vi "Write Config Unitest.vi"(8 "error in (no error)":errorcluster, 11 "main ref":T1) -> (0 "error out":errorcluster)   [LabVIEW 2025]
uses:
  controls/LAB-IQ UI Data.ctl
  Config file  FGV Unitest enum.ctl
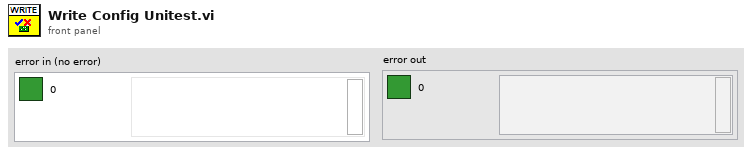
[diagram p1: front panel]
types:
  T1 = typedef "LAB-IQ UI Data.ctl" = cluster{"Main Home Screen":cluster{"GUI":refnum<vi>, "Platform Settings":refnum<vi>, "Configure":refnum<vi>, "Home":refnum<vi>, "EXIT":refnum<vi>, "service 2":refnum<vi>, "MainPage":refnum<vi>, "Analysis":refnum<vi>}, "Platform Settings":cluster{"mm/s  Surge":refnum<vi>, "Update Surge Speed":refnum<vi>, "Drive Error":refnum<vi>, "Disable Axis Jog Soft Limits":refnum<vi>, "mm/s  Sway":refnum<vi>, "Sway and Surge COM Status":refnum<vi>, "Heave COM Status":refnum<vi>, "Enable Platform":refnum<vi>, "Surge Forward Main":refnum<vi>, "Sway Right Main":refnum<vi>, "Sway Left Main":refnum<vi>, "Heave Down Main":refnum<vi>, "Heave Up main":refnum<vi>, "Update Sway Speed":refnum<vi>, "Update Heave Speed":refnum<vi>, "mm/s Heave":refnum<vi>, "mm/sec":refnum<vi>, "mm":refnum<vi>, "Surge Backward Main":refnum<vi>}, "Analysis Screen":cluster{"Analysis Home":refnum<vi>, "Surface Analysis":refnum<vi>, "Imaging":refnum<vi>, "Image Analysis":refnum<vi>, "Post Analysis":refnum<vi>}, "Config Screen":cluster{"Select Load Head":refnum<vi>, "Notes :":refnum<vi>, "FILE":refnum<vi>, "Sample ID :":refnum<vi>, "Operator ID :":refnum<vi>, "Operator Name :":refnum<vi>, "Auto":refnum<vi>}, "Motion Module":cluster{"zNL":refnum<vi>, "NL disp":refnum<vi>, "Rotary Tab":refnum<vi>, "Motion Direction:  3":refnum<vi>, "E.Velocity 2":refnum<vi>, "e.v/ssr 2":refnum<vi>, "Enter Fixed E.Velocity 2":refnum<vi>, "Enter Final SRR 2":refnum<vi>, "Enter initial SRR 2":refnum<vi>, "Enter Fixed SRR 2":refnum<vi>, "Enter the Final E.Velocity (m/s) 2":refnum<vi>, "Enter initial E.Velocity (m/s) 2":refnum<vi>, "Final Speed (RPM) 3":refnum<vi>, "Initial Speed (RPM) 2":refnum<vi>, "Enter the Final Velocity (m/s) 3":refnum<vi>, "Enter initial Velocity (m/s)  3":refnum<vi>, "Ramp Up 2":refnum<vi>, "TEST SELECTION":refnum<vi>, "SPEED SELECTION : ":refnum<vi>, "Angular Oscillation Set":refnum<vi>, "Traction":refnum<vi>, "Step Speed":refnum<vi>, "StepTable For Load-Speed":refnum<vi>, "StepTable For Speed":refnum<vi>, "Surge Forward MM":refnum<vi>, "Surge Backward MM":refnum<vi>, "M3 Image":refnum<vi>, "String 39":refnum<vi>, "Sway Left MM":refnum<vi>, "Sway Right MM":refnum<vi>, "Disable Axis Jog Soft Limits":refnum<vi>, "mm":refnum<vi>, "Heave Down MM":refnum<vi>, "Heave Up MM":refnum<vi>, "Wear Track Diameter (mm)":refnum<vi>, "Set WTD":refnum<vi>, "HomeScratch":refnum<vi>, "HomeRot":refnum<vi>, "PlaceModule":refnum<vi>, "Enter the Angle (Deg)":refnum<vi>, "Enter the Frequency (Hz)":refnum<vi>, "Motion Mode:":refnum<vi>, "LR Sway":refnum<vi>, "Rot Hor":refnum<vi>, "Scratch":refnum<vi>, "LR Cam":refnum<vi>, "MMBack":refnum<vi>, "MMNext":refnum<vi>, "Rot Ver":refnum<vi>, "Rotary Module Selection":refnum<vi>, "calculate rotary":refnum<vi>, "SPEED SELECTION : rotary":refnum<vi>, "Import 2":refnum<vi>, "Save 2":refnum<vi>, "File Path :  2":refnum<vi>, "String 45":refnum<vi>, "StepTable For Speed 3":refnum<vi>, "Enter the Speed(mm/sec)":refnum<vi>, "Enter the Speed(RPM)":refnum<vi>, "Enter Scratch Speed (mm/s):":refnum<vi>, "SwaySpeed Set":refnum<vi>, "Scartch Offset":refnum<vi>, "Motion type:":refnum<vi>, "HomeScratch 2":refnum<vi>, "Enter Scratch length (mm):":refnum<vi>, "Wear Track Diameter":refnum<vi>, "Rotary Speed Exced":refnum<vi>, "Scratch Mode":refnum<vi>, "No of Scratch":refnum<vi>}, "Environmental control":cluster{"Humidity  Status  3":refnum<vi>, "Low Temp  Status  2":refnum<vi>, "TK4 status 2":refnum<vi>, "Stage Temperature":refnum<vi>, "Sample Temperature":refnum<vi>, "Humidity (Amb)":refnum<vi>, "Clear List":refnum<vi>, "Add to list":refnum<vi>, "Wear":refnum<vi>, "Vibration":refnum<vi>, "Humidity (Chamber)":refnum<vi>, "Temperature (Chamber)":refnum<vi>, "ECR ":refnum<vi>, "Temperature (Amb)":refnum<vi>, "Microphone":refnum<vi>, "Acoustic Emission 3":refnum<vi>, "SNext":refnum<vi>, "APBack":refnum<vi>, "Enter the Temperature (°C):":refnum<vi>, "Enter the Stage \nTemperature (°C):":refnum<vi>, "Enter the Humidity (%Rh):":refnum<vi>, "Low Temp":refnum<vi>, "High Temp":refnum<vi>, "Humidity":refnum<vi>, "Sensors Picked":refnum<vi>}, "About Screen":cluster{"Password":refnum<vi>, "Home Service":refnum<vi>, "Advanced Setting":refnum<vi>, "About Tab":refnum<vi>, "ECR Port:":refnum<vi>, "Ramp Port:":refnum<vi>, "Installation/Replacement completed":refnum<vi>, "Loahead":refnum<vi>, "Heave and Surge COM Port:":refnum<vi>, "Sway COM Port:":refnum<vi>, "Temp Modbus:":refnum<vi>, "Humidity Port:":refnum<vi>, "Edit Gain Constants":refnum<vi>, "Save Gain Constants":refnum<vi>}, "Main Screen":cluster{"Main Screen Tab":refnum<vi>, "Angle and Frequency":refnum<vi>, "Stroke (mm)":refnum<vi>, "Angle (Deg)":refnum<vi>, "Main Speed Tab":refnum<vi>, "MTM MOTOR DISPLAY":refnum<vi>, "Disc Speed (m/sec)":refnum<vi>, "Ball Speed (m/sec)":refnum<vi>, "Disc Speed (RPM)":refnum<vi>, "Ball Speed (RPM)":refnum<vi>, "SPEED TAB":refnum<vi>, "Speed (m/sec)":refnum<vi>, "Set Speed (m/sec)":refnum<vi>, "Speed (RPM)":refnum<vi>, "Set Speed":refnum<vi>, "Time Tab":refnum<vi>, "Time ( HH:MM:SS ) 2":refnum<vi>, "Test Duration":refnum<vi>, "Test Duration 4":refnum<vi>, "TEST CYCLE":refnum<vi>, "TOTAL CYCLES":refnum<vi>, "Set Load (N)":refnum<vi>, "Temp Tabs":refnum<vi>, "Heater":refnum<vi>, "TK4 status":refnum<vi>, "ChamberTemp":refnum<vi>, "SetTmp":refnum<vi>, "Controller  Status":refnum<vi>, "ChamberTemp 2":refnum<vi>, "SetTmp 2":refnum<vi>, "Controller  Status 2":refnum<vi>, "ChamberTemp 3":refnum<vi>, "SetTmp 3":refnum<vi>, "Cooling":refnum<vi>, "Load Communication":refnum<vi>, "Ambient \nTemperature":refnum<vi>, "HumCOMStatus":refnum<vi>, "Ambient\n Humidity":refnum<vi>, "Freq (Hz)":refnum<vi>, "Load En":refnum<vi>, "NLt":refnum<vi>, "zNL 2":refnum<vi>, "Humidity On":refnum<vi>, "humidity disp":refnum<vi>, "Set Humidity":refnum<vi>, "NL disp 2":refnum<vi>, "Humidity On 2":refnum<vi>, "humidity disp 2":refnum<vi>, "Set Humidity 2":refnum<vi>, "NL disp 3":refnum<vi>, "AppLoadSeq scratch":refnum<vi>, "Stop Scratch":refnum<vi>, "ClrLog":refnum<vi>, "Trip Log":refnum<vi>, "STOP":refnum<vi>, "Start Test":refnum<vi>, "Test status":refnum<vi>, "AR Led":refnum<vi>, "Data":refnum<vi>, "Health":refnum<vi>, "Sway COM Status":refnum<vi>, "Heave COM Status":refnum<vi>, "Grp Tab":refnum<vi>, "Sub Graph":refnum<vi>, "SD (mm)":refnum<vi>, "Siliding distance Reset Graph":refnum<vi>, "SDGp":refnum<vi>, "Humidity Reset Graph":refnum<vi>, "HumrGp":refnum<vi>, "Acoustic Emission (mV)":refnum<vi>, "Aqucostic Reset Graph":refnum<vi>, "gACQUOS":refnum<vi>, "ECR RESET":refnum<vi>, "ECR":refnum<vi>, "Temperature Reset":refnum<vi>, "Acoustic Emission (mV) 2":refnum<vi>, "Aqucostic Reset Graph 2":refnum<vi>, "gACQUOS 2":refnum<vi>, "ECR RESET 2":refnum<vi>, "ECR 2":refnum<vi>, "Temperature Reset 2":refnum<vi>, "Temperature (deg c)":refnum<vi>, "Speed Reset Graph":refnum<vi>, "Speed Tab":refnum<vi>, "MTM DISC  SPEED":refnum<vi>, "MTM BALL SPEED":refnum<vi>, "speed mm/sec":refnum<vi>, "Hymidity":refnum<vi>, "Humidity Disable trip":refnum<vi>, "CoF Trip  2":refnum<vi>, "Depth Trip":refnum<vi>, "Weart Deapth":refnum<vi>, "Depth Reset Graph":refnum<vi>, "Weart":refnum<vi>, "Depthz":refnum<vi>, "Depth (µm)":refnum<vi>, "WearGp":refnum<vi>, "NL Trip 2":refnum<vi>, "Load pid":refnum<vi>, "Load Disable Trip":refnum<vi>, "Load Reset Graph":refnum<vi>, "NL Display 4":refnum<vi>, "Main Chart 3":refnum<vi>, "BACK":refnum<vi>, "Depth Trip 2":refnum<vi>, "COF TRIP ":refnum<vi>, "Friction Force (N)":refnum<vi>, "FF Reset Graph":refnum<vi>, "FF Disable Trip":refnum<vi>, "FF TRIP":refnum<vi>, "COF Disable Trip":refnum<vi>, "COF Reset Graph":refnum<vi>, "Start Test Temp":refnum<vi>, "zFF":refnum<vi>, "Friction Force (N) Graph":refnum<vi>, "Coefficient of Friction":refnum<vi>, "Scratch Start Test":refnum<vi>, "FF Tab":refnum<vi>, "Cyclic Friction Force (N)":refnum<vi>, "CZ FF":refnum<vi>, "Cyclic Friction Force (N) Graph":refnum<vi>, "Cyclic Coefficient of Friction":refnum<vi>, "Cyclic FF TRIP":refnum<vi>, "Cyclic FF Disable Trip":refnum<vi>, "cyclic COF Disable Trip":refnum<vi>, "cyclic COF TRIP":refnum<vi>, "cyclic COF Reset Graph":refnum<vi>, "Cyclic FF Reset Graph":refnum<vi>, "Test Trip":refnum<vi>, "Multi Scratch Pass":refnum<vi>}, "Loading":cluster{"Indentation":refnum<vi>, "Reference Sample":refnum<vi>, "Load Cell Communication Slide":refnum<vi>, "com 3":refnum<vi>, "com":refnum<vi>, "DecaForce COM Status":refnum<vi>, "Update":refnum<vi>, "Clear 3":refnum<vi>, "seq":refnum<vi>, "Stribeck table":refnum<vi>, "Stribeck Table  For loading":refnum<vi>, "Loading Mode":refnum<vi>, "Enter the Final Load (N)":refnum<vi>, "Enter the CoF Trip":refnum<vi>, "Enter the Friction Force Trip":refnum<vi>, "Enter the Normal load Trip":refnum<vi>, "Enter the Load  (N)":refnum<vi>, "KiloForce":refnum<vi>, "DecaForce ":refnum<vi>, "MicroForce":refnum<vi>, "LHBack":refnum<vi>, "LHNext":refnum<vi>, "Enter the Loading Rate (N/min)":refnum<vi>, "Message":refnum<vi>, "Warning 2":refnum<vi>, "SSP 0.75":refnum<vi>, "SSP 0.5":refnum<vi>, "SSP 0.3":refnum<vi>, "Warning":refnum<vi>, "gui GIF":refnum<vi>, "Communication is established":refnum<vi>, "AppLoad 4":refnum<vi>, "Multipoint":refnum<vi>, "Load Selection":refnum<vi>}, "PID":cluster{"Ramp MulFac":refnum<vi>, "pulses LoadDiffRamp(2..10)":refnum<vi>, "PulseControlRamp(diff<=3N)":refnum<vi>, "SetLoadDeadband(%) Load(0-10N)":refnum<vi>, "PID gains out delay (microForce)":refnum<vi>, "Ramp":refnum<vi>, "Gain 2":refnum<vi>, "pulses LoadDiff(2..10)":refnum<vi>, "pulses LoadDiff(11..50)":refnum<vi>, "PulseControl(diff<=3N)":refnum<vi>, "SetLoadDeadband(%)  2":refnum<vi>, "Dummy Run":refnum<vi>, "Vertical load (N)":refnum<vi>, "AutoTune":refnum<vi>, "Offset 3 ":refnum<vi>, "apply load":refnum<vi>, "Offset  3":refnum<vi>, "apply load 2":refnum<vi>, "Enter ByPass Load":refnum<vi>, "reinit 3":refnum<vi>, "output range delay":refnum<vi>, "PID gains out delay":refnum<vi>, "Bypass Load":refnum<vi>, "pulsesSent":refnum<vi>, "pulses ":refnum<vi>, "actpid":refnum<vi>, "gFF Rot":refnum<vi>, "pulses LoadDiff(21..1000)":refnum<vi>, "Delay":refnum<vi>, "deadband":refnum<vi>}, "Config Parameters":cluster{"Tab Control 3":refnum<vi>, "Tab Control 19":refnum<vi>, "SAMPLES":refnum<vi>, "Re-initilaize":refnum<vi>, "Filter ON/OFF":refnum<vi>, "TracHomeSurgeOffsetCounts 10MM":refnum<vi>, "TracHomeSwayOffsetCounts 10MM":refnum<vi>, "Acoustic Emission:":refnum<vi>, "Apply Filter (FF)":refnum<vi>, "Filter% 2":refnum<vi>, "Apply Filter (Load)":refnum<vi>, "Filter% ":refnum<vi>, "Sway distance (mm)":refnum<vi>, "Surge distance (mm)":refnum<vi>, "DataSavingLoopDelay(ms)":refnum<vi>, "SAVE 2":refnum<vi>, "Enter Distance":refnum<vi>, "Sway Counts:":refnum<vi>, "Distance (mm): 3":refnum<vi>, "Surge Counts:":refnum<vi>, "Distance (mm): 2":refnum<vi>, "Distance (mm):":refnum<vi>, "Heave Counts:":refnum<vi>, "LRMHomeSurgeOffsetCounts":refnum<vi>, "LRMHomeSwayOffsetCounts":refnum<vi>, "TracHomeSurgeOffsetCounts 20MM":refnum<vi>, "TracHomeSwayOffsetCounts 20MM":refnum<vi>, "RotHomeSwayOffsetCounts":refnum<vi>, "RotHomeSurgeOffsetCounts":refnum<vi>, "Heave distance":refnum<vi>, "Zmm":refnum<vi>, "Heave Pulses/mm":refnum<vi>, "Surge Pulses/mm":refnum<vi>, "Sway Pulses/mm":refnum<vi>, "Heave Pitch":refnum<vi>, "Surge Pitch":refnum<vi>, "Sway Pitch":refnum<vi>, "Heave PPR":refnum<vi>, "Surge PPR":refnum<vi>, "Sway PPR":refnum<vi>, "Tab Control 5":refnum<vi>, "Tab Control 14":refnum<vi>, "Tab Control 26":refnum<vi>, "AE":refnum<vi>, "Heave Loop Delay":refnum<vi>, "Heave PID Speed":refnum<vi>, "Surge Jog Speed":refnum<vi>, "Heave Jog Speed":refnum<vi>, "Sway Loop Delay":refnum<vi>, "Sway PID Speed":refnum<vi>, "Sway Jog Speed":refnum<vi>}, "Loading Com Port":cluster{"ClearAll":refnum<vi>, "Mz(Nm)":refnum<vi>, "My(Nm)":refnum<vi>, "Mx(Nm)":refnum<vi>, "Save Dwell":refnum<vi>, "Mx ":refnum<vi>, "My ":refnum<vi>, "Mz":refnum<vi>, "Fx(N)":refnum<vi>, "Fy(N)":refnum<vi>, "Fz(N)":refnum<vi>, "ZeroAll":refnum<vi>, "Acq Delay (ms)":refnum<vi>, "Burst Delay (ms)":refnum<vi>, "model":refnum<vi>, "SN":refnum<vi>, "FFx(N)":refnum<vi>, "Sensor IP":refnum<vi>, "Port":refnum<vi>, "FFy(N)":refnum<vi>, "Load(N)":refnum<vi>, "delete Handle":refnum<vi>, "Create Handle":refnum<vi>, "ft_data":refnum<vi>, "ft_range":refnum<vi>, "ft_data 2":refnum<vi>, "stop 6":refnum<vi>, "running_flag":refnum<vi>, "ft_udp_handle":refnum<vi>, "get-data-return":refnum<vi>, "get-range-return":refnum<vi>, "zero-return":refnum<vi>, "filter-return":refnum<vi>, "initial-return":refnum<vi>, "deleteHandle-result":refnum<vi>, "Load Cell Temp":refnum<vi>}, "Heave AND Surge":cluster{"SURGE POSE":refnum<vi>, "error out Read":refnum<vi>, "HEAVE POSE":refnum<vi>, "State":refnum<vi>, "Homed":refnum<vi>, "Sequence ID":refnum<vi>, "error out Write":refnum<vi>, "faultCode":refnum<vi>, "Ack ID":refnum<vi>, "SPEED":refnum<vi>, "Distance":refnum<vi>, "Mode Command":refnum<vi>, "Heave and Surge Read":refnum<vi>, "Read Heave Temp":refnum<vi>, "Spare 15":refnum<vi>, "Spare 14":refnum<vi>, "Spare 13":refnum<vi>, "Spare 12":refnum<vi>, "Spare 11":refnum<vi>, "Spare 10":refnum<vi>, "Spare 9":refnum<vi>, "Spare 8":refnum<vi>, "Spare 7":refnum<vi>, "Spare 6":refnum<vi>, "Spare 5":refnum<vi>, "Spare 4":refnum<vi>, "Spare 2":refnum<vi>, "Spare 1":refnum<vi>, "Node Id":refnum<vi>, "Spare 3":refnum<vi>, "SPARE 4":refnum<vi>, "SPARE 3":refnum<vi>, "SPARE 2":refnum<vi>, "SPARE 1":refnum<vi>, "fwMajor":refnum<vi>, "fwMinor":refnum<vi>, "Manual Write":refnum<vi>, "Heave and Surge Write":refnum<vi>}, "New PID LOGIC":cluster{"Fine Tune Zone":refnum<vi>, "PID SDelay":refnum<vi>, "Max_pos_limit":refnum<vi>, "Min_pos_limit":refnum<vi>, "i_limit":refnum<vi>, "pct_scale":refnum<vi>, "Deadband":refnum<vi>, "Kd":refnum<vi>, "Ki":refnum<vi>, "Kp":refnum<vi>, "Current Position":refnum<vi>, "Set Load":refnum<vi>, "Current Load":refnum<vi>, "Pulse delta":refnum<vi>, "Init Step":refnum<vi>, "Max Step Linit":refnum<vi>}, "SWAY ":cluster{"fwMajor":refnum<vi>, "Homed":refnum<vi>, "Rotary POSE":refnum<vi>, "State":refnum<vi>, "SWAY POSE":refnum<vi>, "Ack ID":refnum<vi>, "faultCode":refnum<vi>, "Node Id":refnum<vi>, "fwMinor":refnum<vi>, "Spare 6":refnum<vi>, "Spare 5":refnum<vi>, "Spare 4":refnum<vi>, "Spare 3":refnum<vi>, "Spare 2":refnum<vi>, "Spare 1":refnum<vi>, "Spare 7":refnum<vi>, "SPARE  5":refnum<vi>, "error out Write  SWAY ":refnum<vi>, "error out Read SWAY ":refnum<vi>, "Manual Write SWAY ":refnum<vi>, "SWAY WRITE":refnum<vi>, "SPARE  4":refnum<vi>, "SPARE  3":refnum<vi>, "SPARE 2":refnum<vi>, "SPARE 1":refnum<vi>, "Spare 15":refnum<vi>, "Spare 14":refnum<vi>, "Spare 13":refnum<vi>, "Spare 12":refnum<vi>, "Spare 11":refnum<vi>, "Spare 9":refnum<vi>, "Spare 8":refnum<vi>, "SPEED":refnum<vi>, "Distance":refnum<vi>, "Mode Command":refnum<vi>, "Sequence ID":refnum<vi>, "SWAY READ":refnum<vi>, "Spare 10":refnum<vi>, "Read SWAY Temp":refnum<vi>}, "Analysis Screen":cluster{"Analysis Home":refnum<vi>, "Refresh 2":refnum<vi>, "MEAN 4":refnum<vi>, "SD 4":refnum<vi>, "VARIANCE 4":refnum<vi>, "MEAN  3":refnum<vi>, "SD  3":refnum<vi>, "VARIANCE  3":refnum<vi>, "MEAN 2":refnum<vi>, "SD  2":refnum<vi>, "VARIANCE 2":refnum<vi>, "MEAN":refnum<vi>, "SD":refnum<vi>, "VARIANCE":refnum<vi>, "File 4 Discription":refnum<vi>, "OPEN 4":refnum<vi>, "File Name 4":refnum<vi>, "OPEN 3":refnum<vi>, "File 3 Discription":refnum<vi>, "File Name 3":refnum<vi>, "Y-AXIS":refnum<vi>, "X-AXIS":refnum<vi>, "XY Graph":refnum<vi>, "File Name 2":refnum<vi>, "File Name 1":refnum<vi>, "OPEN 2":refnum<vi>, "OPEN 1":refnum<vi>, "File 1 Discription ":refnum<vi>, "File 2 Discription":refnum<vi>}}
  T2 = typedef "Config file  FGV Unitest enum.ctl" = enum16{"OPEN", "READ", "WRITE", "CLOSE"}
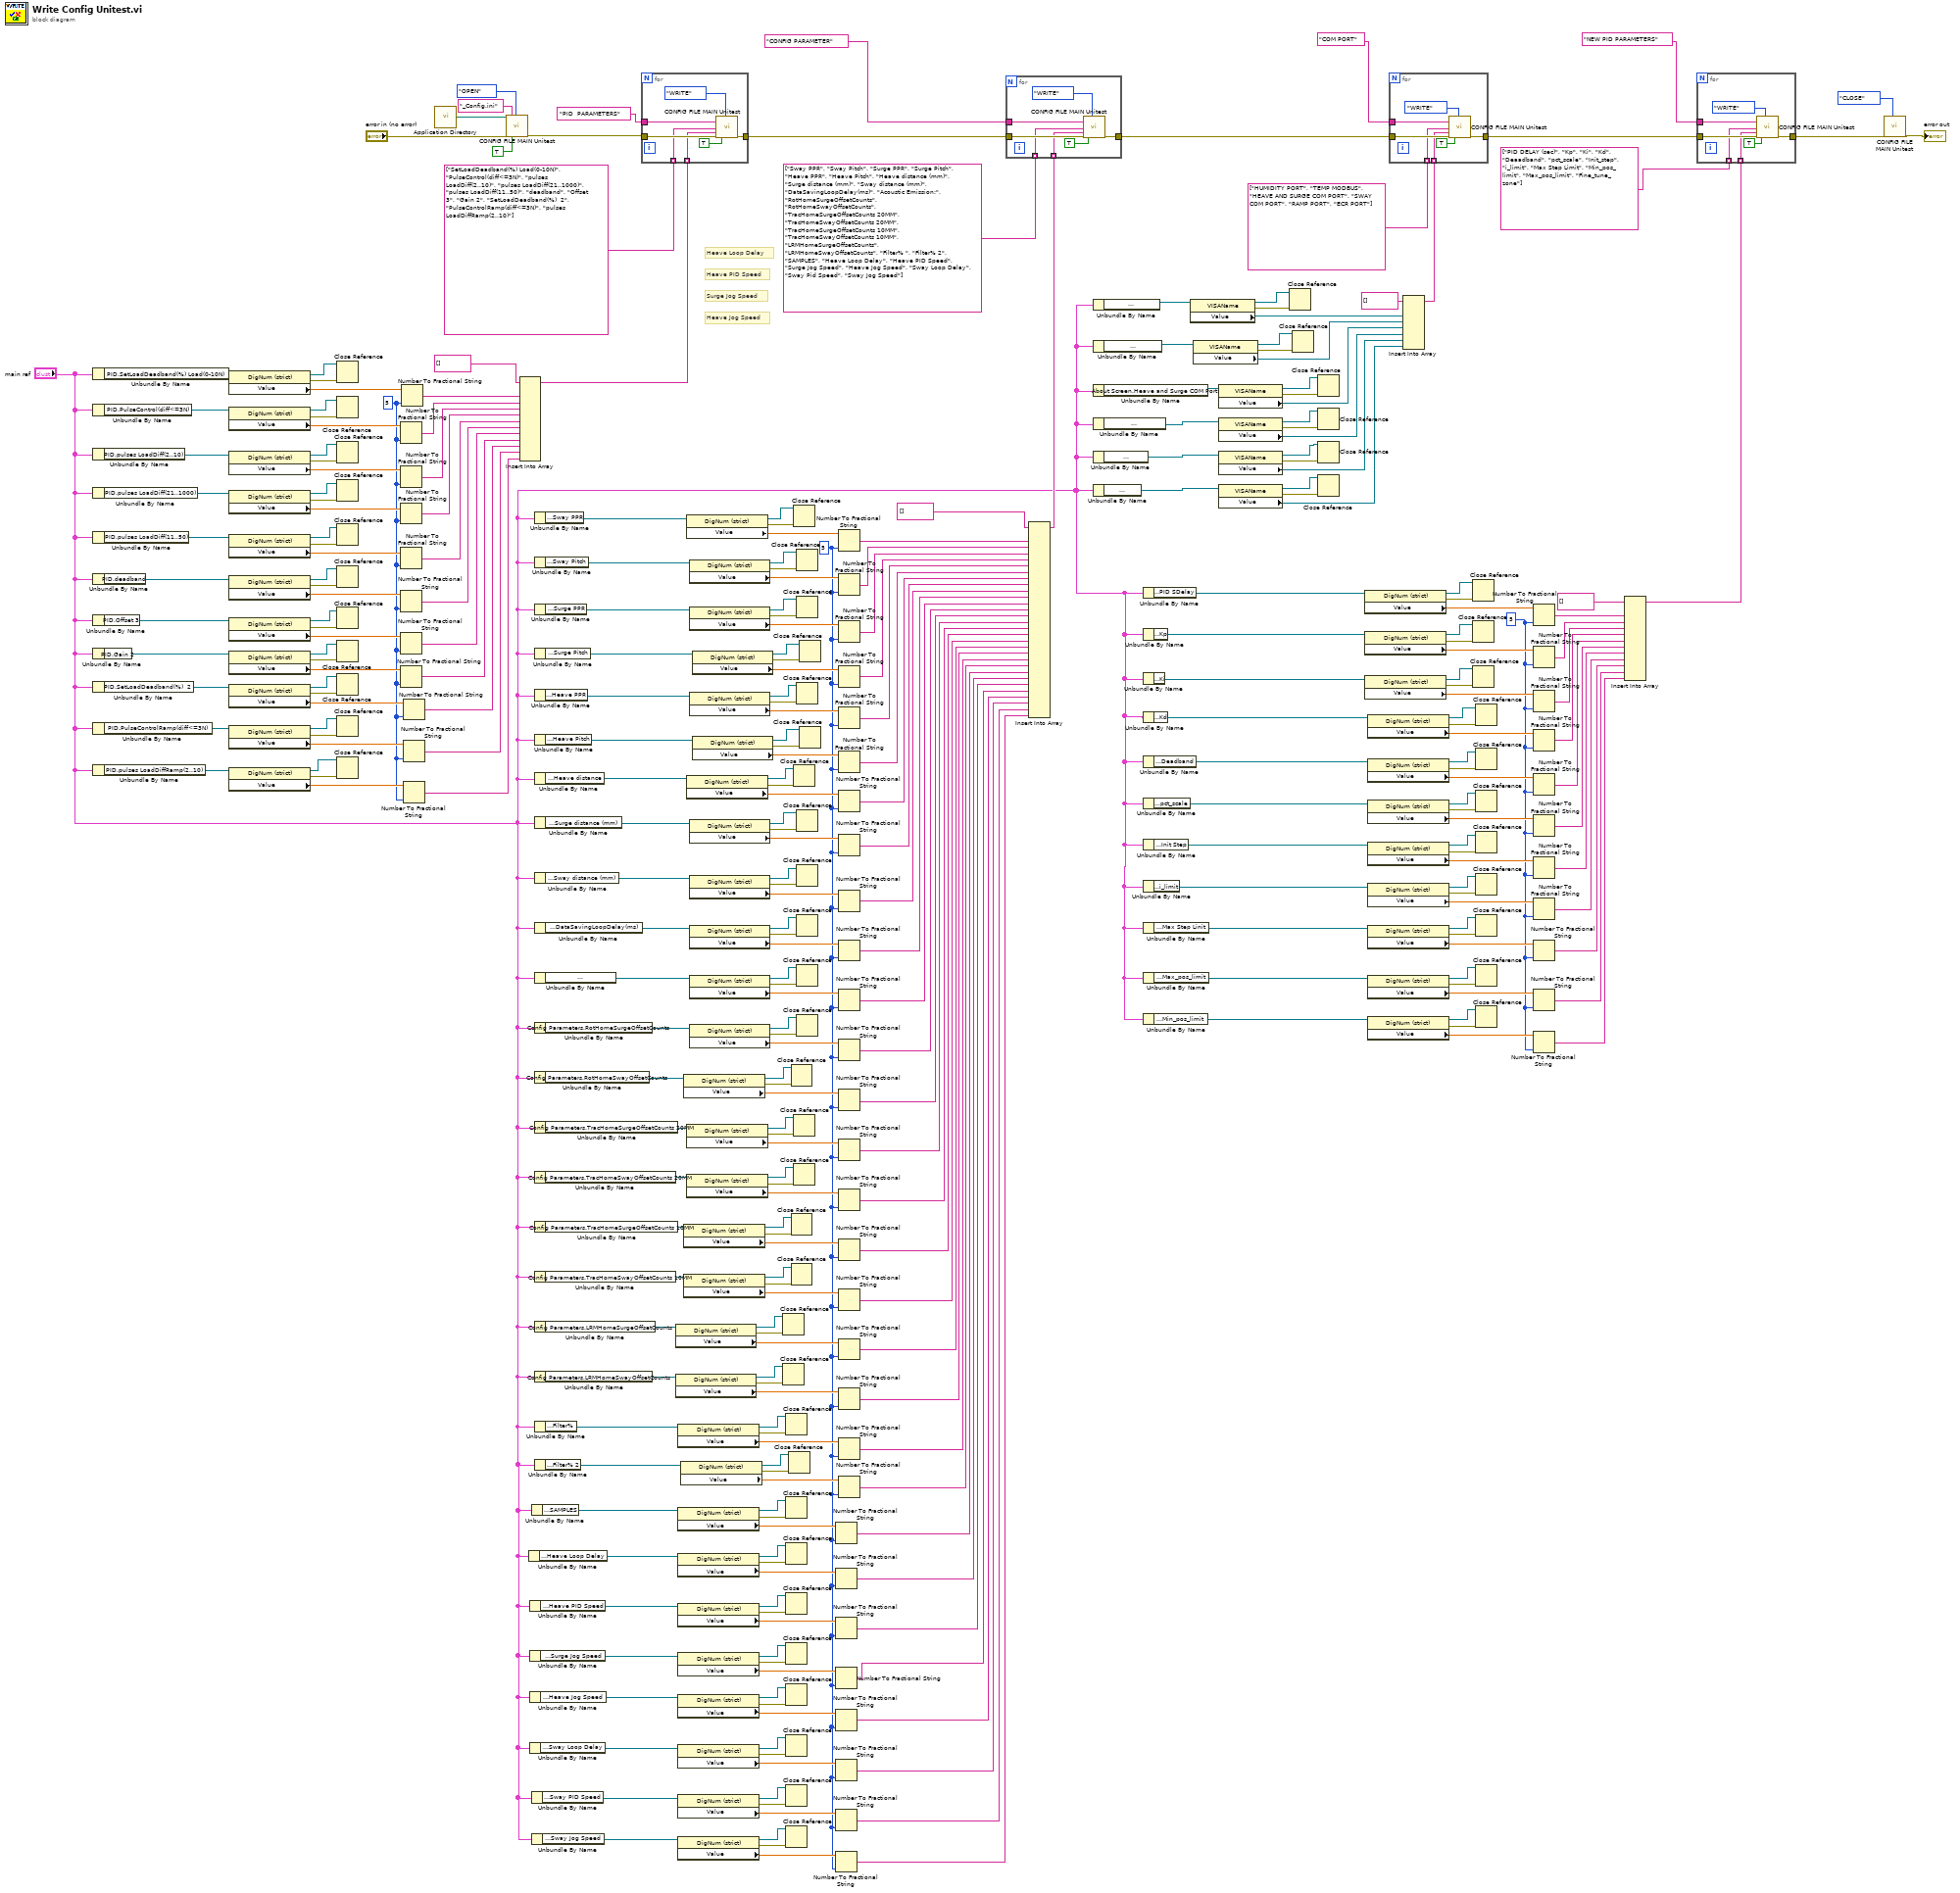
[diagram p0: block diagram]
diagram:
  w31 = i16 5 ("precision (6)")
  w4 = i16 5 ("precision (6)")
  w250 = i16 5 ("precision (6)")
  # "Heave Jog Speed"
  # "Surge Jog Speed"
  # "Heave PID Speed"
  # "Heave Loop Delay"
  n1 = Unbundle By Name("main ref") -> ("PID.SetLoadDeadband(%) Load(0-10N)"=w294:refnum<vi>)
  n2 = Unbundle By Name("main ref") -> ("PID.PulseControl(diff<=3N)"=w289:refnum<vi>)
  n3 = Unbundle By Name("main ref") -> ("PID.pulses LoadDiff(2..10)"=w288:refnum<vi>)
  n4 = Unbundle By Name("main ref") -> ("PID.pulses LoadDiff(21..1000)"=w283:refnum<vi>)
  n5 = Unbundle By Name("main ref") -> ("PID.pulses LoadDiff(11..50)"=w282:refnum<vi>)
  n6 = Unbundle By Name("main ref") -> ("PID.deadband"=w277:refnum<vi>)
  n7 = Unbundle By Name("main ref") -> ("PID.Offset 3"=w276:refnum<vi>)
  n8 = Unbundle By Name("main ref") -> ("PID.Gain 2"=w271:refnum<vi>)
  n9 = Unbundle By Name("main ref") -> ("PID.SetLoadDeadband(%)  2"=w270:refnum<vi>)
  n10 = Unbundle By Name("main ref") -> ("PID.PulseControlRamp(diff<=3N)"=w266:refnum<vi>)
  n11 = Unbundle By Name("main ref") -> ("PID.pulses LoadDiffRamp(2..10)"=w264:refnum<vi>)
  n12 = property class="DigNum (strict)"(reference=w294) -> (reference out=w292:refnum<vi>, error out=w293:errorcluster, "Value"=w260:dbl)  [unwired: 1 in]
  n13 = property class="DigNum (strict)"(reference=w289) -> (reference out=w291:refnum<vi>, error out=w290:errorcluster, "Value"=w261:dbl)  [unwired: 1 in]
  n14 = property class="DigNum (strict)"(reference=w288) -> (reference out=w286:refnum<vi>, error out=w287:errorcluster, "Value"=w259:dbl)  [unwired: 1 in]
  n15 = property class="DigNum (strict)"(reference=w283) -> (reference out=w285:refnum<vi>, error out=w284:errorcluster, "Value"=w258:dbl)  [unwired: 1 in]
  n16 = property class="DigNum (strict)"(reference=w282) -> (reference out=w280:refnum<vi>, error out=w281:errorcluster, "Value"=w257:dbl)  [unwired: 1 in]
  n17 = property class="DigNum (strict)"(reference=w277) -> (reference out=w279:refnum<vi>, error out=w278:errorcluster, "Value"=w256:dbl)  [unwired: 1 in]
  n18 = property class="DigNum (strict)"(reference=w276) -> (reference out=w274:refnum<vi>, error out=w275:errorcluster, "Value"=w255:dbl)  [unwired: 1 in]
  n19 = property class="DigNum (strict)"(reference=w271) -> (reference out=w273:refnum<vi>, error out=w272:errorcluster, "Value"=w254:dbl)  [unwired: 1 in]
  n20 = property class="DigNum (strict)"(reference=w270) -> (reference out=w268:refnum<vi>, error out=w269:errorcluster, "Value"=w253:dbl)  [unwired: 1 in]
  n21 = property class="DigNum (strict)"(reference=w266) -> (reference out=w265:refnum<vi>, error out=w267:errorcluster, "Value"=w252:dbl)  [unwired: 1 in]
  n22 = property class="DigNum (strict)"(reference=w264) -> (reference out=w262:refnum<vi>, error out=w263:errorcluster, "Value"=w251:dbl)  [unwired: 1 in]
  n23 = Close Reference(reference=w292, error in (no error)=w293) -> ()  [unwired: 1 out]
  n24 = Close Reference(reference=w291, error in (no error)=w290) -> ()  [unwired: 1 out]
  n25 = Close Reference(reference=w286, error in (no error)=w287) -> ()  [unwired: 1 out]
  n26 = Close Reference(reference=w285, error in (no error)=w284) -> ()  [unwired: 1 out]
  n27 = Close Reference(reference=w280, error in (no error)=w281) -> ()  [unwired: 1 out]
  n28 = Close Reference(reference=w279, error in (no error)=w278) -> ()  [unwired: 1 out]
  n29 = Close Reference(reference=w274, error in (no error)=w275) -> ()  [unwired: 1 out]
  n30 = Close Reference(reference=w273, error in (no error)=w272) -> ()  [unwired: 1 out]
  n31 = Close Reference(reference=w268, error in (no error)=w269) -> ()  [unwired: 1 out]
  n32 = Close Reference(reference=w265, error in (no error)=w267) -> ()  [unwired: 1 out]
  n33 = Close Reference(reference=w262, error in (no error)=w263) -> ()  [unwired: 1 out]
  n34 = Number To Fractional String(number=w261, precision (6)=w250) -> (F-format string=w247:string)  [unwired: 2 in]
  n35 = Number To Fractional String(number=w259, precision (6)=w250) -> (F-format string=w246:string)  [unwired: 2 in]
  n36 = Number To Fractional String(number=w258, precision (6)=w250) -> (F-format string=w245:string)  [unwired: 2 in]
  n37 = Number To Fractional String(number=w257, precision (6)=w250) -> (F-format string=w244:string)  [unwired: 2 in]
  n38 = Number To Fractional String(number=w256, precision (6)=w250) -> (F-format string=w243:string)  [unwired: 2 in]
  n39 = Number To Fractional String(number=w255, precision (6)=w250) -> (F-format string=w242:string)  [unwired: 2 in]
  n40 = Number To Fractional String(number=w254, precision (6)=w250) -> (F-format string=w241:string)  [unwired: 2 in]
  n41 = Number To Fractional String(number=w260, precision (6)=w250) -> (F-format string=w248:string)  [unwired: 2 in]
  n42 = Number To Fractional String(number=w253, precision (6)=w250) -> (F-format string=w240:string)  [unwired: 2 in]
  n43 = Number To Fractional String(number=w252, precision (6)=w250) -> (F-format string=w239:string)  [unwired: 2 in]
  n44 = Number To Fractional String(number=w251, precision (6)=w250) -> (F-format string=w238:string)  [unwired: 2 in]
  n45 = call <vilib>:"Application Directory.vi"() -> ("Application Directory"=w307:path)
  n46 = call "CONFIG FILE MAIN Unitest.vi"("File Path"=w307, "error in"="error in (no error)", "file name"="_Config.ini", "PARAMETER/CONFIG"=TRUE, "Config Enum"=Config_file__FGV_Unitest_enum."OPEN") -> ("error out"=w306:errorcluster)  [unwired: 13 in, 1 out]
  n47 = Insert Into Array(array=string[] [], new element #1=w248, new element #2=w247, new element #3=w246, new element #4=w245, new element #5=w244, new element #6=w243, new element #7=w242, new element #8=w241, new element #9=w240, new element #10=w239, new element #11=w238) -> (w237:string[])  [unwired: 1 in]
  n48 = Unbundle By Name("main ref") -> ("Config Parameters.Heave Loop Delay"=w96:refnum<vi>)
  n49 = Unbundle By Name("main ref") -> ("Config Parameters.Heave PID Speed"=w95:refnum<vi>)
  n50 = Unbundle By Name("main ref") -> ("Config Parameters.Surge Jog Speed"=w88:refnum<vi>)
  n51 = Unbundle By Name("main ref") -> ("Config Parameters.Heave Jog Speed"=w87:refnum<vi>)
  n52 = Unbundle By Name("main ref") -> ("Config Parameters.Sway Loop Delay"=w6:refnum<vi>)
  n53 = Unbundle By Name("main ref") -> ("Config Parameters.SAMPLES"=w154:refnum<vi>)
  n54 = Unbundle By Name("main ref") -> ("Config Parameters.Sway PID Speed"=w13:refnum<vi>)
  n55 = Unbundle By Name("main ref") -> ("Config Parameters.Sway Jog Speed"=w14:refnum<vi>)
  n56 = Unbundle By Name("main ref") -> ("Config Parameters.Sway PPR"=w236:refnum<vi>)
  n57 = Unbundle By Name("main ref") -> ("Config Parameters.Sway Pitch"=w229:refnum<vi>)
  n58 = Unbundle By Name("main ref") -> ("Config Parameters.Surge PPR"=w221:refnum<vi>)
  n59 = Unbundle By Name("main ref") -> ("Config Parameters.Surge Pitch"=w228:refnum<vi>)
  n60 = Unbundle By Name("main ref") -> ("Config Parameters.Heave PPR"=w220:refnum<vi>)
  n61 = Unbundle By Name("main ref") -> ("Config Parameters.Heave Pitch"=w214:refnum<vi>)
  n62 = Unbundle By Name("main ref") -> ("Config Parameters.Heave distance"=w206:refnum<vi>)
  n63 = Unbundle By Name("main ref") -> ("Config Parameters.Surge distance (mm)"=w212:refnum<vi>)
  n64 = Unbundle By Name("main ref") -> ("Config Parameters.Sway distance (mm)"=w203:refnum<vi>)
  n65 = Unbundle By Name("main ref") -> ("Config Parameters.DataSavingLoopDelay(ms)"=w200:refnum<vi>)
  n66 = Unbundle By Name("main ref") -> ("Config Parameters.Acoustic Emission:"=w195:refnum<vi>)
  n67 = Unbundle By Name("main ref") -> ("Config Parameters.RotHomeSurgeOffsetCounts"=w192:refnum<vi>)
  n68 = Unbundle By Name("main ref") -> ("Config Parameters.RotHomeSwayOffsetCounts"=w187:refnum<vi>)
  n69 = Unbundle By Name("main ref") -> ("Config Parameters.TracHomeSurgeOffsetCounts 20MM"=w184:refnum<vi>)
  n70 = Unbundle By Name("main ref") -> ("Config Parameters.TracHomeSwayOffsetCounts 20MM"=w179:refnum<vi>)
  n71 = Unbundle By Name("main ref") -> ("Config Parameters.TracHomeSurgeOffsetCounts 10MM"=w173:refnum<vi>)
  n72 = Unbundle By Name("main ref") -> ("Config Parameters.TracHomeSwayOffsetCounts 10MM"=w178:refnum<vi>)
  n73 = Unbundle By Name("main ref") -> ("Config Parameters.LRMHomeSurgeOffsetCounts"=w167:refnum<vi>)
  n74 = Unbundle By Name("main ref") -> ("Config Parameters.LRMHomeSwayOffsetCounts"=w162:refnum<vi>)
  n75 = Unbundle By Name("main ref") -> ("Config Parameters.Filter%"=w161:refnum<vi>)
  n76 = Unbundle By Name("main ref") -> ("Config Parameters.Filter% 2"=w155:refnum<vi>)
  n77 = for {
    tunnel: w306 -> [w318]
    tunnel: "PID  PARAMETERS" ("WRITE /READ SECTION") -> [w317]
    tunnel: string[] ["SetLoadDeadband(%) Load(0-10N)", "PulseControl(diff<=3N)", "pulses LoadDiff(2..10)", "pulses LoadDiff(21..1000)", "pulses LoadDiff(11..50)", "deadband", "Offset  3", "Gain 2", "SetLoadDeadband(%)  2", "PulseControlRamp(diff<=3N)", "pulses LoadDiffRamp(2..10)"] -> [w314] mode=indexing
    tunnel: [w316] -> w303
    tunnel: w237 -> [w313] mode=indexing
    n78 = call "CONFIG FILE MAIN Unitest.vi"("WRITE /READ SECTION"=w317, "WRITE KEY"=w314, "WRITE VALUE"=w313, "error in"=w318, "PARAMETER/CONFIG"=TRUE, "Config Enum"=Config_file__FGV_Unitest_enum."WRITE") -> ("error out"=w316:errorcluster)  [unwired: 12 in, 1 out]
  }
  n79 = property class="DigNum (strict)"(reference=w167) -> (reference out=w168:refnum<vi>, error out=w166:errorcluster, "Value"=w165:dbl)  [unwired: 1 in]
  n80 = property class="DigNum (strict)"(reference=w162) -> (reference out=w169:refnum<vi>, error out=w163:errorcluster, "Value"=w164:dbl)  [unwired: 1 in]
  n81 = property class="DigNum (strict)"(reference=w161) -> (reference out=w158:refnum<vi>, error out=w160:errorcluster, "Value"=w159:dbl)  [unwired: 1 in]
  n82 = property class="DigNum (strict)"(reference=w154) -> (reference out=w151:refnum<vi>, error out=w153:errorcluster, "Value"=w152:dbl)  [unwired: 1 in]
  n83 = property class="DigNum (strict)"(reference=w96) -> (reference out=w99:refnum<vi>, error out=w97:errorcluster, "Value"=w98:dbl)  [unwired: 1 in]
  n84 = property class="DigNum (strict)"(reference=w95) -> (reference out=w92:refnum<vi>, error out=w94:errorcluster, "Value"=w93:dbl)  [unwired: 1 in]
  n85 = property class="DigNum (strict)"(reference=w88) -> (reference out=w91:refnum<vi>, error out=w89:errorcluster, "Value"=w90:dbl)  [unwired: 1 in]
  n86 = property class="DigNum (strict)"(reference=w87) -> (reference out=w84:refnum<vi>, error out=w86:errorcluster, "Value"=w85:dbl)  [unwired: 1 in]
  n87 = property class="DigNum (strict)"(reference=w6) -> (reference out=w9:refnum<vi>, error out=w7:errorcluster, "Value"=w8:dbl)  [unwired: 1 in]
  n88 = property class="DigNum (strict)"(reference=w13) -> (reference out=w10:refnum<vi>, error out=w12:errorcluster, "Value"=w11:dbl)  [unwired: 1 in]
  n89 = property class="DigNum (strict)"(reference=w14) -> (reference out=w17:refnum<vi>, error out=w15:errorcluster, "Value"=w16:dbl)  [unwired: 1 in]
  n90 = property class="DigNum (strict)"(reference=w155) -> (reference out=w150:refnum<vi>, error out=w156:errorcluster, "Value"=w157:dbl)  [unwired: 1 in]
  n91 = property class="DigNum (strict)"(reference=w187) -> (reference out=w186:refnum<vi>, error out=w188:errorcluster, "Value"=w189:dbl)  [unwired: 1 in]
  n92 = property class="DigNum (strict)"(reference=w173) -> (reference out=w171:refnum<vi>, error out=w174:errorcluster, "Value"=w175:dbl)  [unwired: 1 in]
  n93 = property class="DigNum (strict)"(reference=w178) -> (reference out=w170:refnum<vi>, error out=w177:errorcluster, "Value"=w176:dbl)  [unwired: 1 in]
  n94 = property class="DigNum (strict)"(reference=w236) -> (reference out=w234:refnum<vi>, error out=w235:errorcluster, "Value"=w233:dbl)  [unwired: 1 in]
  n95 = property class="DigNum (strict)"(reference=w206) -> (reference out=w125:refnum<vi>, error out=w207:errorcluster, "Value"=w208:dbl)  [unwired: 1 in]
  n96 = property class="DigNum (strict)"(reference=w184) -> (reference out=w185:refnum<vi>, error out=w183:errorcluster, "Value"=w182:dbl)  [unwired: 1 in]
  n97 = property class="DigNum (strict)"(reference=w179) -> (reference out=w172:refnum<vi>, error out=w180:errorcluster, "Value"=w181:dbl)  [unwired: 1 in]
  n98 = property class="DigNum (strict)"(reference=w229) -> (reference out=w231:refnum<vi>, error out=w230:errorcluster, "Value"=w232:dbl)  [unwired: 1 in]
  n99 = property class="DigNum (strict)"(reference=w221) -> (reference out=w223:refnum<vi>, error out=w222:errorcluster, "Value"=w224:dbl)  [unwired: 1 in]
  n100 = property class="DigNum (strict)"(reference=w220) -> (reference out=w213:refnum<vi>, error out=w219:errorcluster, "Value"=w218:dbl)  [unwired: 1 in]
  n101 = property class="DigNum (strict)"(reference=w212) -> (reference out=w210:refnum<vi>, error out=w211:errorcluster, "Value"=w209:dbl)  [unwired: 1 in]
  n102 = property class="DigNum (strict)"(reference=w203) -> (reference out=w202:refnum<vi>, error out=w204:errorcluster, "Value"=w205:dbl)  [unwired: 1 in]
  n103 = property class="DigNum (strict)"(reference=w200) -> (reference out=w201:refnum<vi>, error out=w199:errorcluster, "Value"=w198:dbl)  [unwired: 1 in]
  n104 = property class="DigNum (strict)"(reference=w195) -> (reference out=w194:refnum<vi>, error out=w196:errorcluster, "Value"=w197:dbl)  [unwired: 1 in]
  n105 = property class="DigNum (strict)"(reference=w192) -> (reference out=w193:refnum<vi>, error out=w191:errorcluster, "Value"=w190:dbl)  [unwired: 1 in]
  n106 = property class="DigNum (strict)"(reference=w228) -> (reference out=w226:refnum<vi>, error out=w227:errorcluster, "Value"=w225:dbl)  [unwired: 1 in]
  n107 = property class="DigNum (strict)"(reference=w214) -> (reference out=w216:refnum<vi>, error out=w215:errorcluster, "Value"=w217:dbl)  [unwired: 1 in]
  n108 = Close Reference(reference=w168, error in (no error)=w166) -> ()  [unwired: 1 out]
  n109 = Close Reference(reference=w169, error in (no error)=w163) -> ()  [unwired: 1 out]
  n110 = Close Reference(reference=w158, error in (no error)=w160) -> ()  [unwired: 1 out]
  n111 = Close Reference(reference=w151, error in (no error)=w153) -> ()  [unwired: 1 out]
  n112 = Close Reference(reference=w99, error in (no error)=w97) -> ()  [unwired: 1 out]
  n113 = Close Reference(reference=w92, error in (no error)=w94) -> ()  [unwired: 1 out]
  n114 = Close Reference(reference=w91, error in (no error)=w89) -> ()  [unwired: 1 out]
  n115 = Close Reference(reference=w84, error in (no error)=w86) -> ()  [unwired: 1 out]
  n116 = Close Reference(reference=w9, error in (no error)=w7) -> ()  [unwired: 1 out]
  n117 = Close Reference(reference=w10, error in (no error)=w12) -> ()  [unwired: 1 out]
  n118 = Close Reference(reference=w17, error in (no error)=w15) -> ()  [unwired: 1 out]
  n119 = Close Reference(reference=w150, error in (no error)=w156) -> ()  [unwired: 1 out]
  n120 = Close Reference(reference=w186, error in (no error)=w188) -> ()  [unwired: 1 out]
  n121 = Close Reference(reference=w171, error in (no error)=w174) -> ()  [unwired: 1 out]
  n122 = Close Reference(reference=w170, error in (no error)=w177) -> ()  [unwired: 1 out]
  n123 = Close Reference(reference=w234, error in (no error)=w235) -> ()  [unwired: 1 out]
  n124 = Close Reference(reference=w125, error in (no error)=w207) -> ()  [unwired: 1 out]
  n125 = Close Reference(reference=w185, error in (no error)=w183) -> ()  [unwired: 1 out]
  n126 = Close Reference(reference=w172, error in (no error)=w180) -> ()  [unwired: 1 out]
  n127 = Close Reference(reference=w231, error in (no error)=w230) -> ()  [unwired: 1 out]
  n128 = Close Reference(reference=w223, error in (no error)=w222) -> ()  [unwired: 1 out]
  n129 = Close Reference(reference=w213, error in (no error)=w219) -> ()  [unwired: 1 out]
  n130 = Close Reference(reference=w210, error in (no error)=w211) -> ()  [unwired: 1 out]
  n131 = Close Reference(reference=w202, error in (no error)=w204) -> ()  [unwired: 1 out]
  n132 = Close Reference(reference=w201, error in (no error)=w199) -> ()  [unwired: 1 out]
  n133 = Close Reference(reference=w194, error in (no error)=w196) -> ()  [unwired: 1 out]
  n134 = Close Reference(reference=w193, error in (no error)=w191) -> ()  [unwired: 1 out]
  n135 = Close Reference(reference=w226, error in (no error)=w227) -> ()  [unwired: 1 out]
  n136 = Close Reference(reference=w216, error in (no error)=w215) -> ()  [unwired: 1 out]
  n137 = Number To Fractional String(number=w152, precision (6)=w4) -> (F-format string=w127:string)  [unwired: 2 in]
  n138 = Number To Fractional String(number=w98, precision (6)=w4) -> (F-format string=w83:string)  [unwired: 2 in]
  n139 = Number To Fractional String(number=w93, precision (6)=w4) -> (F-format string=w82:string)  [unwired: 2 in]
  n140 = Number To Fractional String(number=w90, precision (6)=w4) -> (F-format string=w81:string)  [unwired: 2 in]
  n141 = Number To Fractional String(number=w85, precision (6)=w4) -> (F-format string=w80:string)  [unwired: 2 in]
  n142 = Number To Fractional String(number=w8, precision (6)=w4) -> (F-format string=w3:string)  [unwired: 2 in]
  n143 = Number To Fractional String(number=w11, precision (6)=w4) -> (F-format string=w2:string)  [unwired: 2 in]
  n144 = Number To Fractional String(number=w16, precision (6)=w4) -> (F-format string=w1:string)  [unwired: 2 in]
  n145 = Number To Fractional String(number=w233, precision (6)=w4) -> (F-format string=w148:string)  [unwired: 2 in]
  n146 = Number To Fractional String(number=w232, precision (6)=w4) -> (F-format string=w147:string)  [unwired: 2 in]
  n147 = Number To Fractional String(number=w224, precision (6)=w4) -> (F-format string=w146:string)  [unwired: 2 in]
  n148 = Number To Fractional String(number=w225, precision (6)=w4) -> (F-format string=w145:string)  [unwired: 2 in]
  n149 = Number To Fractional String(number=w218, precision (6)=w4) -> (F-format string=w144:string)  [unwired: 2 in]
  n150 = Number To Fractional String(number=w217, precision (6)=w4) -> (F-format string=w143:string)  [unwired: 2 in]
  n151 = Number To Fractional String(number=w208, precision (6)=w4) -> (F-format string=w142:string)  [unwired: 2 in]
  n152 = Number To Fractional String(number=w209, precision (6)=w4) -> (F-format string=w141:string)  [unwired: 2 in]
  n153 = Number To Fractional String(number=w205, precision (6)=w4) -> (F-format string=w140:string)  [unwired: 2 in]
  n154 = Number To Fractional String(number=w198, precision (6)=w4) -> (F-format string=w139:string)  [unwired: 2 in]
  n155 = Number To Fractional String(number=w197, precision (6)=w4) -> (F-format string=w138:string)  [unwired: 2 in]
  n156 = Number To Fractional String(number=w190, precision (6)=w4) -> (F-format string=w137:string)  [unwired: 2 in]
  n157 = Number To Fractional String(number=w189, precision (6)=w4) -> (F-format string=w136:string)  [unwired: 2 in]
  n158 = Number To Fractional String(number=w182, precision (6)=w4) -> (F-format string=w135:string)  [unwired: 2 in]
  n159 = Number To Fractional String(number=w181, precision (6)=w4) -> (F-format string=w134:string)  [unwired: 2 in]
  n160 = Number To Fractional String(number=w175, precision (6)=w4) -> (F-format string=w133:string)  [unwired: 2 in]
  n161 = Number To Fractional String(number=w176, precision (6)=w4) -> (F-format string=w132:string)  [unwired: 2 in]
  n162 = Number To Fractional String(number=w165, precision (6)=w4) -> (F-format string=w131:string)  [unwired: 2 in]
  n163 = Number To Fractional String(number=w164, precision (6)=w4) -> (F-format string=w130:string)  [unwired: 2 in]
  n164 = Number To Fractional String(number=w159, precision (6)=w4) -> (F-format string=w129:string)  [unwired: 2 in]
  n165 = Number To Fractional String(number=w157, precision (6)=w4) -> (F-format string=w128:string)  [unwired: 2 in]
  n166 = Insert Into Array(array=string[] [], new element #1=w148, new element #2=w147, new element #3=w146, new element #4=w145, new element #5=w144, new element #6=w143, new element #7=w142, new element #8=w141, new element #9=w140, new element #10=w139, new element #11=w138, new element #12=w137, new element #13=w136, new element #14=w135, new element #15=w134, new element #16=w133, new element #17=w132, new element #18=w131, new element #19=w130, new element #20=w129, new element #21=w128, new element #22=w127, new element #23=w83, new element #24=w82, new element #25=w81, new element #26=w80, new element #27=w3, new element #28=w2, new element #29=w1) -> (w126:string[])  [unwired: 1 in]
  n167 = for {
    tunnel: w303 -> [w325]
    tunnel: "CONFIG PARAMETER" ("WRITE /READ SECTION") -> [w324]
    tunnel: [w323] -> w300
    tunnel: string[] ["Sway PPR", "Sway Pitch", "Surge PPR", "Surge Pitch", "Heave PPR", "Heave Pitch", "Heave distance (mm)", "Surge distance (mm)", "Sway distance (mm)", "DataSavingLoopDelay(ms)", "Acoustic Emission:", "RotHomeSurgeOffsetCounts", "RotHomeSwayOffsetCounts", "TracHomeSurgeOffsetCounts 20MM", "TracHomeSwayOffsetCounts 20MM", "TracHomeSurgeOffsetCounts 10MM", "TracHomeSwayOffsetCounts 10MM", "LRMHomeSurgeOffsetCounts", "LRMHomeSwayOffsetCounts", "Filter% ", "Filter% 2", "SAMPLES", "Heave Loop Delay", "Heave PID Speed", "Surge Jog Speed", "Heave Jog Speed", "Sway Loop Delay", "Sway Pid Speed", "Sway Jog Speed"] -> [w321] mode=indexing
    tunnel: w126 -> [w319] mode=indexing
    n168 = call "CONFIG FILE MAIN Unitest.vi"("WRITE /READ SECTION"=w324, "WRITE KEY"=w321, "WRITE VALUE"=w319, "error in"=w325, "PARAMETER/CONFIG"=TRUE, "Config Enum"=Config_file__FGV_Unitest_enum."WRITE") -> ("error out"=w323:errorcluster)  [unwired: 12 in, 1 out]
  }
  n169 = Unbundle By Name("main ref") -> ("About Screen.Humidity Port:"=w123:refnum<vi>)
  n170 = Unbundle By Name("main ref") -> ("About Screen.Temp Modbus:"=w118:refnum<vi>)
  n171 = Unbundle By Name("main ref") -> ("About Screen.Heave and Surge COM Port:"=w115:refnum<vi>)
  n172 = Unbundle By Name("main ref") -> ("About Screen.Sway COM Port:"=w111:refnum<vi>)
  n173 = Unbundle By Name("main ref") -> ("About Screen.Ramp Port:"=w110:refnum<vi>)
  n174 = Unbundle By Name("main ref") -> ("About Screen.ECR Port:"=w107:refnum<vi>)
  n175 = Unbundle By Name("main ref") -> ("New PID LOGIC.PID SDelay"=w73:refnum<vi>)
  n176 = Unbundle By Name("main ref") -> ("New PID LOGIC.Kp"=w72:refnum<vi>)
  n177 = Unbundle By Name("main ref") -> ("New PID LOGIC.Ki"=w67:refnum<vi>)
  n178 = Unbundle By Name("main ref") -> ("New PID LOGIC.Kd"=w66:refnum<vi>)
  n179 = Unbundle By Name("main ref") -> ("New PID LOGIC.Deadband"=w62:refnum<vi>)
  n180 = Unbundle By Name("main ref") -> ("New PID LOGIC.pct_scale"=w61:refnum<vi>)
  n181 = Unbundle By Name("main ref") -> ("New PID LOGIC.Init Step"=w58:refnum<vi>)
  n182 = Unbundle By Name("main ref") -> ("New PID LOGIC.i_limit"=w57:refnum<vi>)
  n183 = Unbundle By Name("main ref") -> ("New PID LOGIC.Max Step Linit"=w54:refnum<vi>)
  n184 = Unbundle By Name("main ref") -> ("New PID LOGIC.Max_pos_limit"=w52:refnum<vi>)
  n185 = Unbundle By Name("main ref") -> ("New PID LOGIC.Min_pos_limit"=w51:refnum<vi>)
  n186 = property class="VISAName"(reference=w123) -> (reference out=w121:refnum<vi>, error out=w122:errorcluster, "Value"=w117:refnum<visa-resource-name>)  [unwired: 1 in]
  n187 = property class="VISAName"(reference=w118) -> (reference out=w120:refnum<vi>, error out=w119:errorcluster, "Value"=w116:refnum<visa-resource-name>)  [unwired: 1 in]
  n188 = property class="VISAName"(reference=w115) -> (reference out=w113:refnum<vi>, error out=w114:errorcluster, "Value"=w106:refnum<visa-resource-name>)  [unwired: 1 in]
  n189 = property class="VISAName"(reference=w111) -> (reference out=w105:refnum<vi>, error out=w112:errorcluster, "Value"=w104:refnum<visa-resource-name>)  [unwired: 1 in]
  n190 = property class="VISAName"(reference=w110) -> (reference out=w101:refnum<vi>, error out=w109:errorcluster, "Value"=w103:refnum<visa-resource-name>)  [unwired: 1 in]
  n191 = property class="VISAName"(reference=w107) -> (reference out=w100:refnum<vi>, error out=w108:errorcluster, "Value"=w102:refnum<visa-resource-name>)  [unwired: 1 in]
  n192 = Close Reference(reference=w121, error in (no error)=w122) -> ()  [unwired: 1 out]
  n193 = Close Reference(reference=w120, error in (no error)=w119) -> ()  [unwired: 1 out]
  n194 = Close Reference(reference=w113, error in (no error)=w114) -> ()  [unwired: 1 out]
  n195 = Close Reference(reference=w105, error in (no error)=w112) -> ()  [unwired: 1 out]
  n196 = Close Reference(reference=w101, error in (no error)=w109) -> ()  [unwired: 1 out]
  n197 = Close Reference(reference=w100, error in (no error)=w108) -> ()  [unwired: 1 out]
  n198 = property class="DigNum (strict)"(reference=w73) -> (reference out=w75:refnum<vi>, error out=w74:errorcluster, "Value"=w42:dbl)  [unwired: 1 in]
  n199 = property class="DigNum (strict)"(reference=w72) -> (reference out=w70:refnum<vi>, error out=w71:errorcluster, "Value"=w41:dbl)  [unwired: 1 in]
  n200 = property class="DigNum (strict)"(reference=w67) -> (reference out=w69:refnum<vi>, error out=w68:errorcluster, "Value"=w40:dbl)  [unwired: 1 in]
  n201 = property class="DigNum (strict)"(reference=w66) -> (reference out=w64:refnum<vi>, error out=w65:errorcluster, "Value"=w39:dbl)  [unwired: 1 in]
  n202 = property class="DigNum (strict)"(reference=w62) -> (reference out=w48:refnum<vi>, error out=w63:errorcluster, "Value"=w38:dbl)  [unwired: 1 in]
  n203 = property class="DigNum (strict)"(reference=w61) -> (reference out=w49:refnum<vi>, error out=w60:errorcluster, "Value"=w37:dbl)  [unwired: 1 in]
  n204 = property class="DigNum (strict)"(reference=w58) -> (reference out=w47:refnum<vi>, error out=w59:errorcluster, "Value"=w36:dbl)  [unwired: 1 in]
  n205 = property class="DigNum (strict)"(reference=w57) -> (reference out=w46:refnum<vi>, error out=w56:errorcluster, "Value"=w35:dbl)  [unwired: 1 in]
  n206 = property class="DigNum (strict)"(reference=w54) -> (reference out=w45:refnum<vi>, error out=w55:errorcluster, "Value"=w34:dbl)  [unwired: 1 in]
  n207 = property class="DigNum (strict)"(reference=w52) -> (reference out=w44:refnum<vi>, error out=w53:errorcluster, "Value"=w33:dbl)  [unwired: 1 in]
  n208 = property class="DigNum (strict)"(reference=w51) -> (reference out=w43:refnum<vi>, error out=w50:errorcluster, "Value"=w32:dbl)  [unwired: 1 in]
  n209 = Insert Into Array(array=string[] [], new element #1=w117, new element #2=w116, new element #3=w106, new element #4=w104, new element #5=w103, new element #6=w102) -> (w296:string[])  [unwired: 1 in]
  n210 = for {
    tunnel: w300 -> [w332]
    tunnel: "COM PORT" ("WRITE /READ SECTION") -> [w331]
    tunnel: [w330] -> w77
    tunnel: string[] ["HUMIDITY PORT", "TEMP MODBUS", "HEAVE AND SURGE COM PORT", "SWAY COM PORT", "RAMP PORT", "ECR PORT"] -> [w328] mode=indexing
    tunnel: w296 -> [w327] mode=indexing
    n211 = call "CONFIG FILE MAIN Unitest.vi"("WRITE /READ SECTION"=w331, "WRITE KEY"=w328, "WRITE VALUE"=w327, "error in"=w332, "PARAMETER/CONFIG"=TRUE, "Config Enum"=Config_file__FGV_Unitest_enum."WRITE") -> ("error out"=w330:errorcluster)  [unwired: 12 in, 1 out]
  }
  n212 = Close Reference(reference=w75, error in (no error)=w74) -> ()  [unwired: 1 out]
  n213 = Close Reference(reference=w70, error in (no error)=w71) -> ()  [unwired: 1 out]
  n214 = Close Reference(reference=w69, error in (no error)=w68) -> ()  [unwired: 1 out]
  n215 = Close Reference(reference=w64, error in (no error)=w65) -> ()  [unwired: 1 out]
  n216 = Close Reference(reference=w48, error in (no error)=w63) -> ()  [unwired: 1 out]
  n217 = Close Reference(reference=w49, error in (no error)=w60) -> ()  [unwired: 1 out]
  n218 = Close Reference(reference=w47, error in (no error)=w59) -> ()  [unwired: 1 out]
  n219 = Close Reference(reference=w46, error in (no error)=w56) -> ()  [unwired: 1 out]
  n220 = Close Reference(reference=w45, error in (no error)=w55) -> ()  [unwired: 1 out]
  n221 = Close Reference(reference=w44, error in (no error)=w53) -> ()  [unwired: 1 out]
  n222 = Close Reference(reference=w43, error in (no error)=w50) -> ()  [unwired: 1 out]
  n223 = Number To Fractional String(number=w42, precision (6)=w31) -> (F-format string=w29:string)  [unwired: 2 in]
  n224 = Number To Fractional String(number=w41, precision (6)=w31) -> (F-format string=w28:string)  [unwired: 2 in]
  n225 = Number To Fractional String(number=w40, precision (6)=w31) -> (F-format string=w27:string)  [unwired: 2 in]
  n226 = Number To Fractional String(number=w39, precision (6)=w31) -> (F-format string=w26:string)  [unwired: 2 in]
  n227 = Number To Fractional String(number=w38, precision (6)=w31) -> (F-format string=w25:string)  [unwired: 2 in]
  n228 = Number To Fractional String(number=w37, precision (6)=w31) -> (F-format string=w24:string)  [unwired: 2 in]
  n229 = Number To Fractional String(number=w36, precision (6)=w31) -> (F-format string=w23:string)  [unwired: 2 in]
  n230 = Number To Fractional String(number=w35, precision (6)=w31) -> (F-format string=w22:string)  [unwired: 2 in]
  n231 = Number To Fractional String(number=w34, precision (6)=w31) -> (F-format string=w21:string)  [unwired: 2 in]
  n232 = Number To Fractional String(number=w33, precision (6)=w31) -> (F-format string=w20:string)  [unwired: 2 in]
  n233 = Number To Fractional String(number=w32, precision (6)=w31) -> (F-format string=w19:string)  [unwired: 2 in]
  n234 = Insert Into Array(array=string[] [], new element #1=w29, new element #2=w28, new element #3=w27, new element #4=w26, new element #5=w25, new element #6=w24, new element #7=w23, new element #8=w22, new element #9=w21, new element #10=w20, new element #11=w19) -> (w18:string[])  [unwired: 1 in]
  n235 = for {
    tunnel: w77 -> [w339]
    tunnel: "NEW PID PARAMETERS" ("WRITE /READ SECTION") -> [w338]
    tunnel: [w337] -> w78
    tunnel: string[] ["PID DELAY (sec)", "Kp", "Ki", "Kd", "Deaadband", "pct_scale", "Init_step", "i_limit", "Max Step Limit", "Min_pos_limit", "Max_pos_limit", "Fine_tune_zone"] -> [w335] mode=indexing
    tunnel: w18 -> [w333] mode=indexing
    n236 = call "CONFIG FILE MAIN Unitest.vi"("WRITE /READ SECTION"=w338, "WRITE KEY"=w335, "WRITE VALUE"=w333, "error in"=w339, "PARAMETER/CONFIG"=TRUE, "Config Enum"=Config_file__FGV_Unitest_enum."WRITE") -> ("error out"=w337:errorcluster)  [unwired: 12 in, 1 out]
  }
  n237 = call "CONFIG FILE MAIN Unitest.vi"("error in"=w78, "Config Enum"=Config_file__FGV_Unitest_enum."CLOSE") -> ("error out"=→"error out":errorcluster)  [unwired: 16 in, 1 out]
